vi "Reward Pulse.vi"(7 "Pulse duration (ms)":dbl, 9 "DO Task":refnum<k21>="BlueSimple_DO") -> ()   [LabVIEW 2010]
uses:
  Controls/Bits to Write.ctl
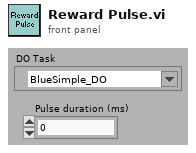
[diagram p1: front panel]
types:
  T1 = typedef "Bits to Write.ctl" = enum16{"LED 1 on", "LED 1 off", "LED 2 on", "LED 2 off", "LED 3 on", "LED 3 off", "LED 4 on", "LED 4 off", "All LEDs on", "All LEDs off", "In trial on", "In trial off", "Buzzer on", "Buzzer off", "Reward on", "Reward off", "Target number", "Trial type preQ on", "Trial type preQ off", "Error on", "Error off", "Trial number", "DBS on", "DBS off", "Sine on", "Sine off", "All Bits On", "All Bits Off", "Init", "Specify mask/pattern"}
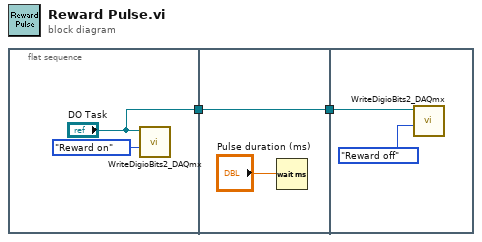
[diagram p0: block diagram]
diagram:
  n1 = flat-sequence {
    tunnel: ["DO Task"] -> w2
    tunnel: w2 -> [w5]
    tunnel: [w5] -> w1
    tunnel: w1 -> [w8]
    frame #0 {
      n2 = call "WriteDigioBits2_DAQmx.vi"("Bits to write"=Bits_to_Write."Reward on", "DO Task"="DO Task") -> ()  [unwired: 9 in, 1 out]
    }
    frame #1 {
      n3 = Wait (ms)(milliseconds to wait="Pulse duration (ms)") -> ()  [unwired: 1 out]
    }
    frame #2 {
      n4 = call "WriteDigioBits2_DAQmx.vi"("Bits to write"=Bits_to_Write."Reward off", "DO Task"=w8) -> ()  [unwired: 9 in, 1 out]
    }
  }
